vi "test_libssh2_session_disconnect.vi"() -> ()   [LabVIEW 2017, in "integration_tests.lvlib"]
uses:
  integration_tests.lvlib
  libssh2/libssh2_session_handshake_tcp.vi
  libssh2/libssh2_init_default.vi
  libssh2/libssh2_session_init_ex.vi
  <vilib>/Utility/tcp.llb/TCP Get Raw Net Object.vi
  libssh2/libssh2_session_handshake_socket.vi
  libssh2/libssh2_session_disconnect_ex.vi
  libssh2/libssh2.lvlib
  support/support.lvlib
  <vilib>/PNR/Transparent Assertions/Transparent Assertions/Transparent Assertions.lvlib
panel:
  out "error out":errorcluster
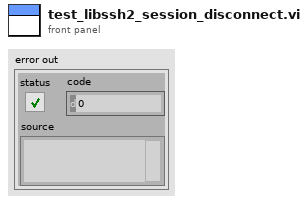
[diagram p1: front panel]
types:
  T1 = typedef "libssh2.lvlib/Session Refnum.ctl" = refnum<k1>
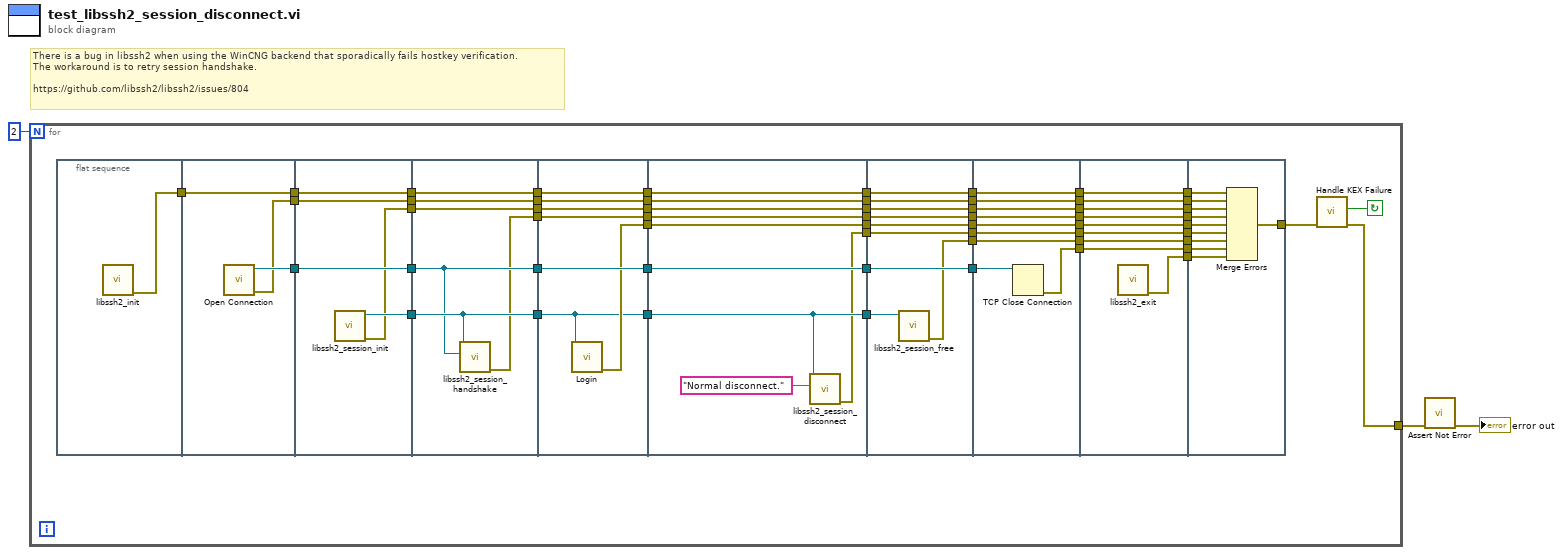
[diagram p0: block diagram]
diagram:
  # "There is a bug in libssh2 when using the WinCNG backend that sporadically fails hostkey verification.\nThe workaround is to retry session handshake.\n\nhttps://github.com/libssh2/libssh2/issues/804"
  n1 = for {
    N: 2 -> [_]
    tunnel: [w8] -> w2
    stop <- w9 continue-if-true
    n2 = flat-sequence {
      tunnel: [w62] -> w61
      tunnel: [w65] -> w60
      tunnel: w61 -> [w64]
      tunnel: [w64] -> w59
      tunnel: [w63] -> w58
      tunnel: w60 -> [w70]
      tunnel: [w70] -> w57
      tunnel: w59 -> [w69]
      tunnel: [w69] -> w56
      tunnel: w58 -> [w68]
      tunnel: [w68] -> w55
      tunnel: [w67] -> w54
      tunnel: [w66] -> w53
      tunnel: w57 -> [w72]
      tunnel: [w72] -> w52
      tunnel: w56 -> [w76]
      tunnel: [w76] -> w51
      tunnel: w55 -> [w75]
      tunnel: [w75] -> w50
      tunnel: [w74] -> w49
      tunnel: w54 -> [w74]
      tunnel: w53 -> [w73]
      tunnel: [w73] -> w48
      tunnel: [w71] -> w47
      tunnel: w52 -> [w83]
      tunnel: [w83] -> w46
      tunnel: w51 -> [w82]
      tunnel: [w82] -> w45
      tunnel: w50 -> [w81]
      tunnel: [w81] -> w44
      tunnel: w49 -> [w77]
      tunnel: w48 -> [w80]
      tunnel: [w80] -> w43
      tunnel: w47 -> [w79]
      tunnel: [w79] -> w42
      tunnel: [w78] -> w41
      tunnel: [w77] -> w40
      tunnel: w46 -> [w92]
      tunnel: [w92] -> w39
      tunnel: w45 -> [w91]
      tunnel: [w91] -> w38
      tunnel: w44 -> [w90]
      tunnel: [w90] -> w37
      tunnel: w43 -> [w89]
      tunnel: [w89] -> w36
      tunnel: w42 -> [w88]
      tunnel: [w88] -> w35
      tunnel: w41 -> [w87]
      tunnel: [w87] -> w34
      tunnel: w40 -> [w86]
      tunnel: [w86] -> w33
      tunnel: [w84] -> w7
      tunnel: w39 -> [w101]
      tunnel: [w101] -> w32
      tunnel: w38 -> [w100]
      tunnel: [w100] -> w31
      tunnel: w37 -> [w99]
      tunnel: [w99] -> w30
      tunnel: w36 -> [w98]
      tunnel: [w98] -> w29
      tunnel: w35 -> [w97]
      tunnel: [w97] -> w28
      tunnel: w34 -> [w96]
      tunnel: [w96] -> w27
      tunnel: [w95] -> w26
      tunnel: w33 -> [w94]
      tunnel: w7 -> [w93]
      tunnel: [w93] -> w6
      tunnel: w32 -> [w110]
      tunnel: w31 -> [w109]
      tunnel: [w109] -> w25
      tunnel: w30 -> [w108]
      tunnel: [w108] -> w24
      tunnel: [w107] -> w23
      tunnel: w29 -> [w106]
      tunnel: [w106] -> w22
      tunnel: w28 -> [w105]
      tunnel: [w105] -> w21
      tunnel: w27 -> [w104]
      tunnel: [w104] -> w20
      tunnel: [w103] -> w19
      tunnel: w26 -> [w103]
      tunnel: w6 -> [w102]
      tunnel: [w102] -> w5
      tunnel: w25 -> [w119]
      tunnel: [w119] -> w18
      tunnel: w24 -> [w118]
      tunnel: [w118] -> w17
      tunnel: w23 -> [w117]
      tunnel: [w117] -> w16
      tunnel: [w116] -> w15
      tunnel: w22 -> [w115]
      tunnel: [w115] -> w14
      tunnel: w21 -> [w114]
      tunnel: [w114] -> w13
      tunnel: w20 -> [w113]
      tunnel: [w113] -> w12
      tunnel: [w112] -> w11
      tunnel: w19 -> [w112]
      tunnel: w5 -> [w111]
      tunnel: [w111] -> w4
      tunnel: w18 -> [w129]
      tunnel: w17 -> [w128]
      tunnel: w16 -> [w127]
      tunnel: w15 -> [w126]
      tunnel: w14 -> [w125]
      tunnel: w13 -> [w124]
      tunnel: w12 -> [w123]
      tunnel: w11 -> [w122]
      tunnel: [w121] -> w10
      tunnel: w4 -> [w120]
      frame #0 {
        n3 = call-poly "libssh2_init.vi"() -> ("error out"=w62:errorcluster)  [unwired: 11 in]
      }
      frame #1 {
        n4 = call "Open Connection.vi"() -> ("error out"=w63:errorcluster, "connection ID"=w65:refnum<k5>)  [unwired: 10 in]
      }
      frame #2 {
        n5 = call "libssh2_session_init.vi"() -> ("error out"=w66:errorcluster, "session"=w67:T1)  [unwired: 10 in]
      }
      frame #3 {
        n6 = call-poly "libssh2_session_handshake.vi"("tcp connection"=w72, "session"=w74) -> ("error out"=w71:errorcluster)  [unwired: 9 in]
      }
      frame #4 {
        n7 = call "Login.vi"("session"=w77) -> ("error out"=w78:errorcluster)  [unwired: 10 in]
      }
      frame #5 {
        n8 = call "libssh2_session_disconnect.vi"("description"="Normal disconnect.", "session"=w86) -> ("error out"=w84:errorcluster)  [unwired: 9 in]
      }
      frame #6 {
        n9 = call "libssh2_session_free.vi"("session"=w94) -> ("error out"=w95:errorcluster)  [unwired: 10 in]
      }
      frame #7 {
        n10 = TCP Close Connection(connection ID=w110) -> (error out=w107:errorcluster)  [unwired: 2 in, 1 out]
      }
      frame #8 {
        n11 = call "libssh2_exit.vi"() -> ("error out"=w116:errorcluster)  [unwired: 11 in]
      }
      frame #9 {
        n12 = Merge Errors(w129, w128, w125, w124, w123, w120, w122, w127, w126) -> (w121:errorcluster)
      }
    }
    n13 = call "Handle KEX Failure.vi"("error in (no error)"=w10) -> ("error out"=w8:errorcluster, "KEX Failure"=w9:bool)  [unwired: 9 in]
  }
  n14 = call <vilib>:"Assert Not Error.vi"("error in (no error)"=w2) -> ("error out"=→"error out":errorcluster)  [unwired: 10 in]
